vi "Sequence name to file name.vi"(7 "Sequence name":string, 11 "error in (no error)":errorcluster) -> (8 "Sequence file path":path, 15 "error out":errorcluster)   [LabVIEW 2011]
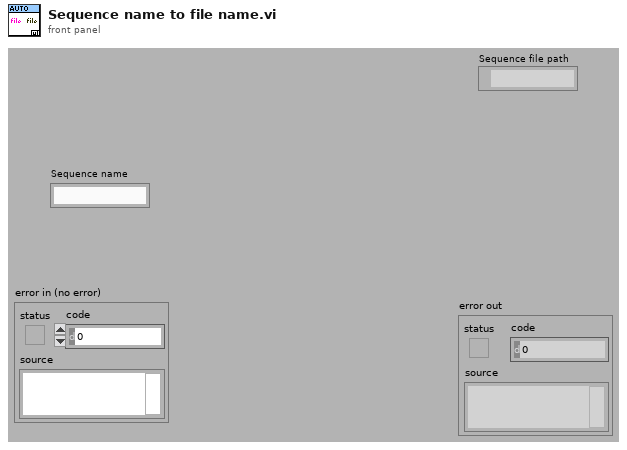
[diagram p1: front panel]
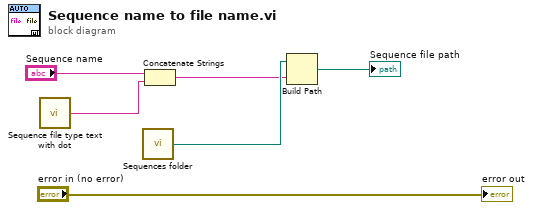
[diagram p0: block diagram]
diagram:
  n1 = call "Sequence file type text with dot.vi"() -> ("Sequrncefile type with dot"=w3:string)  [unwired: 14 in, 1 out]
  n2 = call "Sequences folder.vi"() -> ("Sequence folder"=w5:path)  [unwired: 14 in, 1 out]
  n3 = Concatenate Strings("Sequence name", w3) -> (w4:string)
  n4 = Build Path(base path=w5, name or relative path=w4) -> (appended path=→"Sequence file path":path)
  "error out" <- "error in (no error)"
